vi "Configure Frequency.vi"(0 "Register Bus":T1, 1 "scope":string(combo)="rx", 5 "LO source":string(combo)="LO1" caption="LO Source", 7 "LO frequency [Hz]":dbl=-1.0 caption="LO Frequency [Hz]" format="%#.3pHz", 9 "frequency [Hz]":dbl=2450000000.0 caption="Frequency [Hz]" format="%#.3pHz", 11 "error in":errorcluster) -> (4 "Register Bus (out)":T1, 6 "coerced LO frequency [Hz]":dbl caption="Coerced LO Frequency [Hz]" format="%#.3pHz", 15 "error out":errorcluster)   [LabVIEW 2017]
doc: "Configures the DSP frequency shift and the mixer (RF up/down-coverter) by enabling the LO, setting the LO frequency, configuring the LO filter, and making any necessary routes.\n\n<B>Input Parameters</B>\n\n<B>Register Bus</B> The Register Bus object created by the ni579x Open VI and used as the session handle for the NI-579x Configuration Design Library.\n\n<B>scope</B> is the channel to configure frequency for. The options are \"rx\" and \"tx\".\n\n<B>LO source</B> is the source of the local oscillator used by the specified mixer. \"LO1\" for the internal LO. \"LO In\" to use an external LO source.\n\n<B>LO frequency [Hz]</B> is the frequency to tune the local oscillator to. The default value of -1 means to set the LO to the value of the 'Frequency [Hz]' input. If the value is not -1, the LO will be set to that value, and the difference between the 'Frequency [Hz]' and the 'LO Frequency [Hz]' will be handled by the DSP.\n\n<B>frequency [Hz]</B> is the requested center frequency for the device.\n\n<B>error in</B> describes error conditions that occur before this node runs. This input provides standard 'error in' functionality.\n\n<B>Output Parameters</B>\n\n<B>Register Bus (out)</B> The Register Bus object created by the ni579x Open VI and used as the session handle for the NI-579x Configuration Design Library.\n\n<B>coerced LO frequency [Hz]</B> is the actual frequency the local oscillator was tuned to.\n\n<B>error out</B> contains error information. This output provides standard 'error out' functionality."
uses:
  <instrlib>/_niInstr/Register Bus/v0/Host/Public/Register Bus Session.ctl
  <instrlib>/_niInstr/Register Bus/v0/Host/Private/Session Data.ctl
  Rx FPGA VI Reference.ctl
  Tx FPGA VI Reference.ctl
  <vilib>/Utility/error.llb/Error Cluster From Error Code.vi
  <vilib>/rvi/errors/niLvFpgaAdjustHostInterfaceError.vi
  <vilib>/rvi/interface/nirviReadWriteControl/nirviReadWriteControl.xnode
  <instrlib>/ni579x/Config/v2/Host/ni579x Config v2 Host.lvlib
  NiFpgaLv.dll
  <vilib>/rvi/interface/Simulation/niFpgaSimulationCallBeginRW.vi
  <instrlib>/_niInstr/Register Bus/v0/Host/niInstr Register Bus v0 Host.lvlib
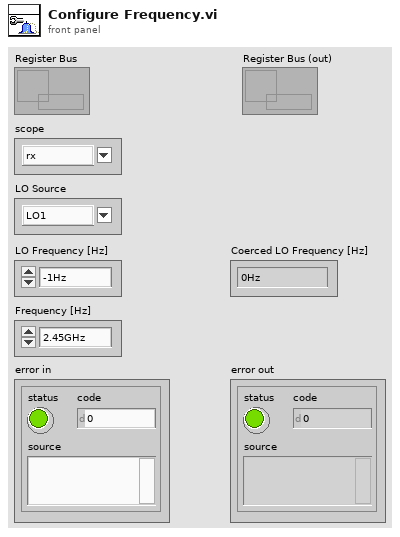
[diagram p1: front panel]
types:
  T1 = typedef "niInstr Register Bus v0 Host.lvlib/Register Bus Session.ctl" = refnum<queue>
  T2 = typedef "Rx FPGA VI Reference.ctl" = refnum<k20>
  T3 = typedef "Tx FPGA VI Reference.ctl" = refnum<k20>
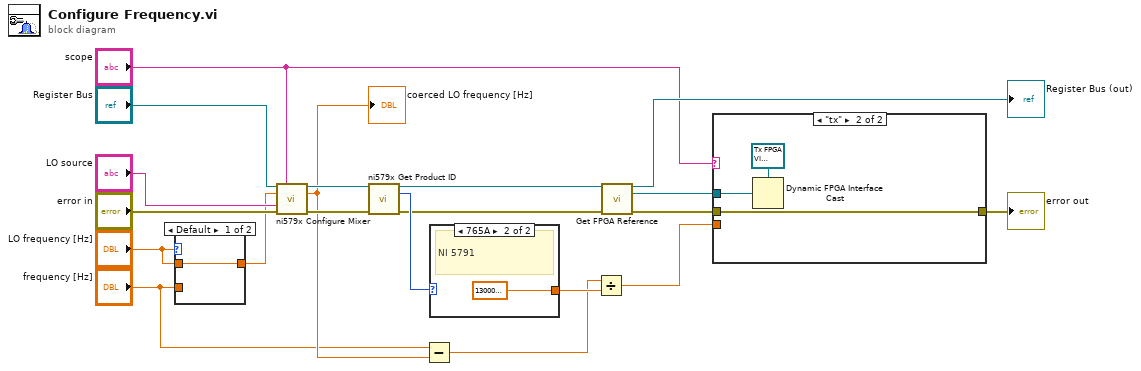
[diagram p0: block diagram]
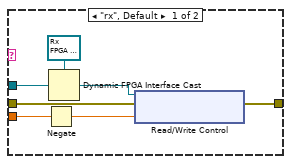
[diagram p3: hidden frame]
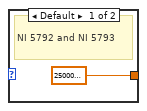
[diagram p4: hidden frame]
diagram:
  n1 = case shown="Default" "LO frequency [Hz]" {
    tunnel: "frequency [Hz]" -> [_ w22]
    tunnel: [w21 w22] -> w3
    tunnel: "LO frequency [Hz]" -> [w21 _]
    frame Default {
    }
    frame -1 {
    }
  }
  n2 = call <instrlib>:"ni579x Configure Mixer.vi"("Register Bus"="Register Bus", "scope"="scope", "frequency [Hz]"=w3, "LO source"="LO source", "Error In"="error in") -> ("Register Bus (out)"=w11:T1, "coerced frequency [Hz]"=w5:dbl, "Error Out"=w10:errorcluster)  [unwired: 8 in]
  "coerced LO frequency [Hz]" <- w5
  n3 = call <instrlib>:"ni579x Get Product ID.vi"("Register Bus"=w11, "Error In"=w10) -> ("Register Bus (out)"=w8:T1, "product ID"=w13:u16, "Error Out"=w9:errorcluster)  [unwired: 11 in]
  n4 = Subtract(x="frequency [Hz]", y=w5) -> (x-y=w7:dbl)
  n5 = case shown="765A" w13 {
    tunnel: [250000000.0 ("clock rate [Hz]") 130000000.0 ("clock rate [Hz]")] -> w12
    frame Default {
      # "NI 5792 and NI 5793"
    }
    frame 30298 {
      # "NI 5791"
    }
  }
  n6 = Divide(x=w7, y=w12) -> (x/y=w20:dbl)
  n7 = call <instrlib>:"Get FPGA Reference.vi"("session in"=w8, "error in"=w9) -> ("session out"=→"Register Bus (out)":T1, "fpga ref"=w19:refnum<k20>, "error out"=w17:errorcluster)  [unwired: 11 in]
  n8 = case shown="\"tx\"" "scope" {
    tunnel: w20 -> [w31 _]
    tunnel: w19 -> [w30 w34]
    tunnel: [w27 w32] -> w18
    tunnel: w17 -> [w26 w32]
    frame "rx", Default {
      n9 = Negate(x=w31) -> (-x=w25:dbl)
      n10 = Dynamic FPGA Interface Cast(Session In=T2 refnum ("FPGA VI Reference Out"), Type=w30) -> (Session Out=w28:T2)
      n11 = xnode "Read/Write Control"("FPGA VI Reference In"=w28, "error in"=w26, "rx.frequency shift"=w25) -> ("error out"=w27:errorcluster)  [unwired: 1 out]
    }
    frame "tx" {
      n12 = Dynamic FPGA Interface Cast(Session In=T3 refnum ("FPGA VI Reference Out"), Type=w34) -> ()  [unwired: 1 out]
    }
  }
  "error out" <- w18
